vi "Read MongoDB.Server.vi"(8 "error in (no error)":errorcluster, 11 "MongoDB.Client in":refnum<class "MongoDB.Client.lvclass">) -> (0 "error out":errorcluster, 2 "MongoDB.Server":refnum<k24>, 3 "MongoDB.Client out":refnum<class "MongoDB.Client.lvclass">)   [LabVIEW 2014, in "MongoDB.Client.lvclass"]
uses:
  MongoDB.Client.lvclass
  C:/Users/Richard/Documents/GitHub/mongo-labview-driver/CSharp/bin/MongoDB.Driver.Legacy.dll
  CSharp/bin/MongoDB.Driver.Legacy.dll
  MongoDB.Client.lvclass/MongoDB.Client.ctl
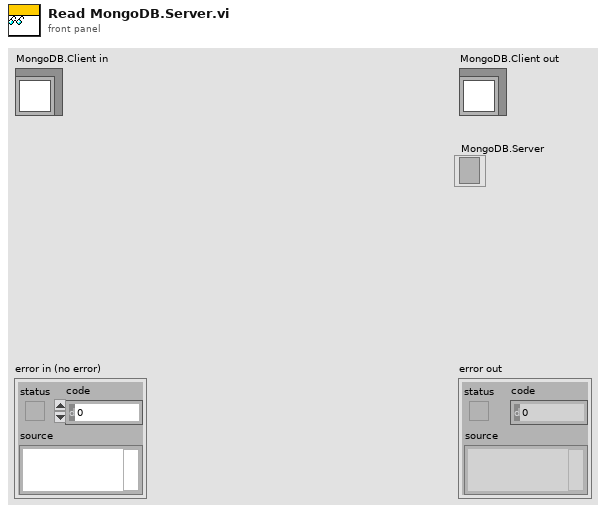
[diagram p1: front panel]
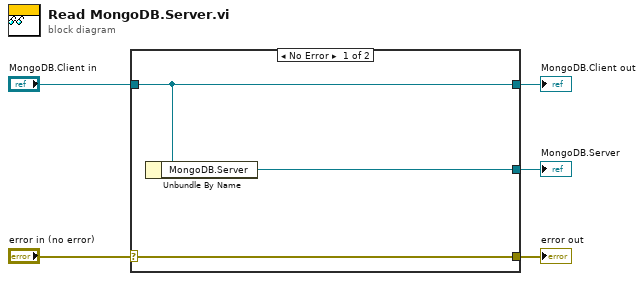
[diagram p0: block diagram]
diagram:
  n1 = case shown="No Error" "error in (no error)" {
    selector: "error in (no error)" -> [w8 w9]
    tunnel: [w8 w9] -> w4
    tunnel: [w7 w10] -> w2
    tunnel: "MongoDB.Client in" -> [w7 w10]
    tunnel: [w6 _] -> w1
    frame No Error {
      n2 = Unbundle By Name(w7) -> ("MongoDB.Server"=w6:refnum<k24>)
    }
    frame Error {
    }
  }
  "error out" <- w4
  "MongoDB.Client out" <- w2
  "MongoDB.Server" <- w1
